vi "Create Channel Array.vi"(8 "error in":errorcluster, 11 "Oscilloscope in":refnum<class "Oscilloscope.lvclass">) -> (0 "error out":errorcluster, 3 "Oscilloscope out":refnum<class "Oscilloscope.lvclass">)   [LabVIEW 2019, in "Oscilloscope.lvlib" / "Oscilloscope.lvclass"]
uses:
  Oscilloscope.lvclass
  Custom Controls/Channel Settings.ctl
  Custom Controls/Vertical Coupling.ctl
  Oscilloscope.lvclass/Oscilloscope.ctl
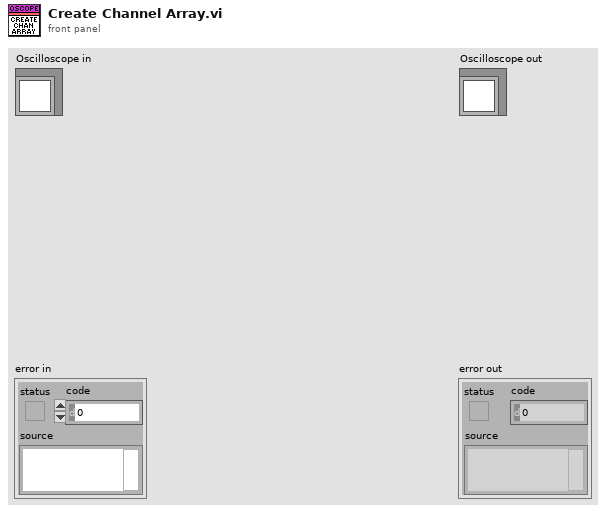
[diagram p1: front panel]
types:
  T1 = typedef "Oscilloscope.lvlib/Oscilloscope.lvclass/Channel Settings.ctl" = cluster{"Amplitude":dbl, "Vertical Coupling":T2, "Probe Attenuation":dbl, "Enable?":bool, "Maximum Input Frequency":dbl, "Input Impedance":u16, "Timeout (s)":dbl}
  T2 = typedef "Oscilloscope.lvlib/Oscilloscope.lvclass/Vertical Coupling.ctl" = enum16{"AC", "DC", "Ground"}
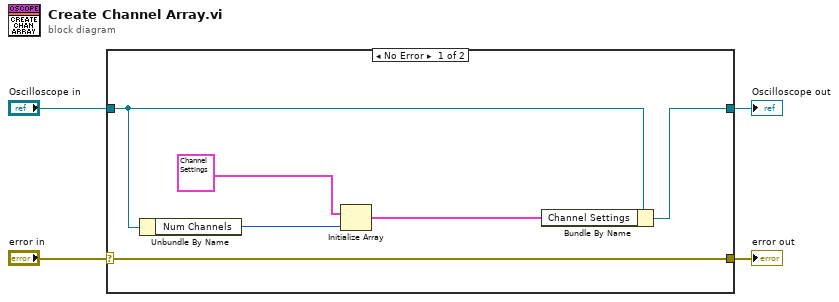
[diagram p0: block diagram]
diagram:
  n1 = case shown="No Error" "error in" {
    selector: "error in" -> [w10 w12]
    tunnel: [w10 w12] -> w3
    tunnel: [w9 w11] -> w1
    tunnel: "Oscilloscope in" -> [w8 w11]
    frame No Error {
      n2 = Unbundle By Name(w8) -> ("Num Channels"=w7:i32)
      n3 = Initialize Array(T1 {"Amplitude"=5.0, "Vertical Coupling"=enum."DC", "Probe Attenuation"=10.0, "Enable?"=FALSE, "Maximum Input Frequency"=15000.0, "Input Impedance"=1, "Timeout (s)"=5.0} ("Channel Settings"), w7) -> (w6:T1[])
      n4 = Bundle By Name(cluster=w8, "Channel Settings"=w6) -> (w9:refnum<class "Oscilloscope.lvclass">)
    }
    frame Error {
    }
  }
  "error out" <- w3
  "Oscilloscope out" <- w1
